vi "Send Event Data Message.vi"(7 "Message Priority (Normal)":T2=enum."Normal", 8 "error in (no error)":errorcluster, 9 "EventFilter Reference":T1, 10 "EventDataMessage":refnum<class "EventDataMessage.lvclass">, 11 "Message Enqueuer in":refnum<class "Message Enqueuer.lvclass">) -> (0 "error out":errorcluster, 3 "Filtered EventDataMessage":refnum<class "EventDataMessage.lvclass">)   [LabVIEW 2017, in "ActorEvents.lvlib" / "EventDataMessage.lvclass"]
doc: "<License>\nCopyright © 2017 Composed Systems, LLC | All rights reserved\nwww.composed.io\n\nAuthor: Ethan Stern <ethan.stern@composed.io>\n\nThis software is provided \"AS IS\" WITHOUT WARRANTIES, either express or implied, AND IS FOR EDUCATIONAL PURPOSES ONLY.\n</License>"
uses:
  EventDataMessage.lvclass
  C:/Program Files (x86)/National Instruments/LabVIEW 2017/vi.lib/ActorFramework/Message/Message.lvclass
  <vilib>/ActorFramework/Message Enqueuer/Message Enqueuer.lvclass
  <vilib>/ActorFramework/Message Enqueuer/Message Priority.ctl
  IEventFilter/EventFilter Reference.ctl
  IEventFilter/IEventFilter.lvclass
  EventDataMessage.lvclass/EventDataMessage.ctl
  <vilib>/ActorFramework/Message Enqueuer/Message Enqueuer.lvclass/Message Enqueuer.ctl
  <vilib>/ActorFramework/Message Priority Queue/Priority Enqueue.vi
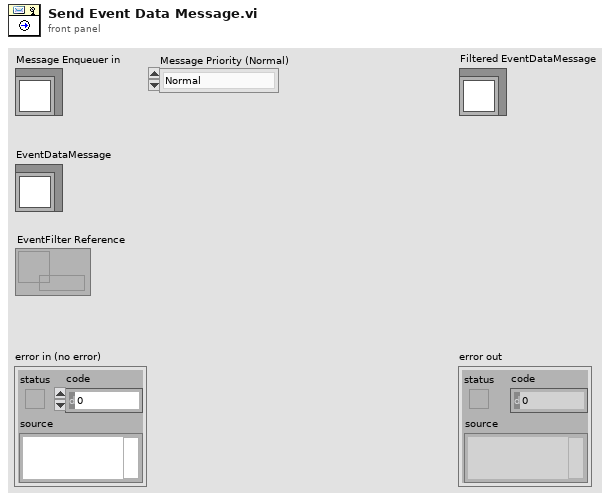
[diagram p1: front panel]
types:
  T1 = typedef "ActorEvents.lvlib/IEventFilter.lvclass/EventFilter Reference.ctl" = refnum<data-value>
  T2 = typedef "Actor Framework.lvlib/Message Enqueuer.lvclass/Message Priority.ctl" = enum16{"Low", "Normal", "High"}
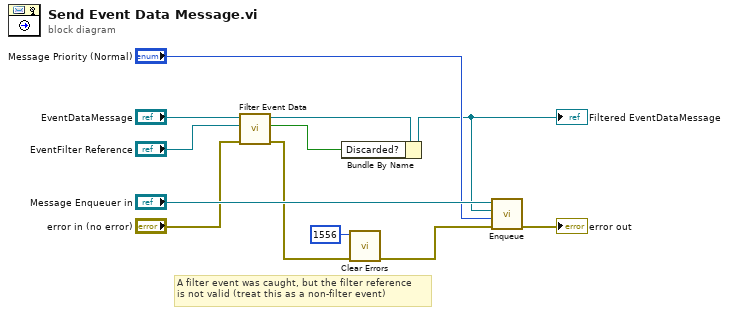
[diagram p0: block diagram]
diagram:
  # "A filter event was caught, but the filter reference\nis not valid (treat this as a non-filter event)"
  n1 = call-dynamic "Filter Event Data.vi"("error in (no error)"="error in (no error)", "EventFilter Reference"="EventFilter Reference", "EventDataMessage in"="EventDataMessage") -> ("error out"=w4:errorcluster, "Discard?"=w5:bool, "EventDataMessage out"=w3:refnum<class "EventDataMessage.lvclass">)  [unwired: 6 in]
  n2 = Bundle By Name(cluster=w3, "Discarded?"=w5) -> (w6:refnum<class "EventDataMessage.lvclass">)
  "Filtered EventDataMessage" <- w6
  n3 = call <vilib>:"Clear Errors.vi"("error in (no error)"=w4, "specific error code to clear (0: all)"=1556) -> ("error out"=w2:errorcluster)  [unwired: 4 in, 1 out]
  n4 = call <vilib>:"Enqueue.vi"("error in (no error)"=w2, "Message Priority (Normal)"="Message Priority (Normal)", "Message"=w6, "Message Enqueuer in"="Message Enqueuer in") -> ("error out"=→"error out":errorcluster)  [unwired: 6 in, 1 out]
